vi "MSScript_Act_Execution.vi"(8 "error in (no error)":errorcluster, 11 "MSScript in":refnum<class "MSScript.lvclass">) -> (0 "error out":errorcluster, 3 "MSScript out":refnum<class "MSScript.lvclass">)   [LabVIEW 2018, in "MSScript.lvclass"]
uses:
  MSScript.lvclass
  MSScript.lvclass/MSScript.ctl
  MSScript_Error_(6002)UndefinedSentence.vi
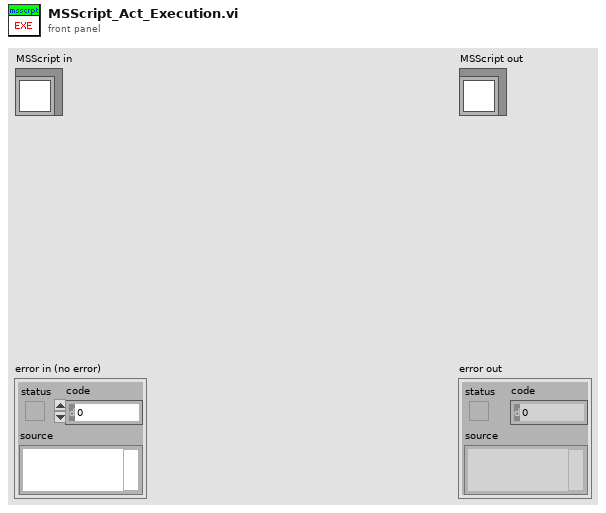
[diagram p1: front panel]
types:
  T1 = cluster{"Type":string, "NAME":cluster{"STR":string, "Start":i32}, "PARAMs":cluster{"STR":string, "Start":i32}[]}[]
  T2 = cluster{"Type":string, "NAME":cluster{"STR":string, "Start":i32}, "PARAMs":cluster{"STR":string, "Start":i32}[]}
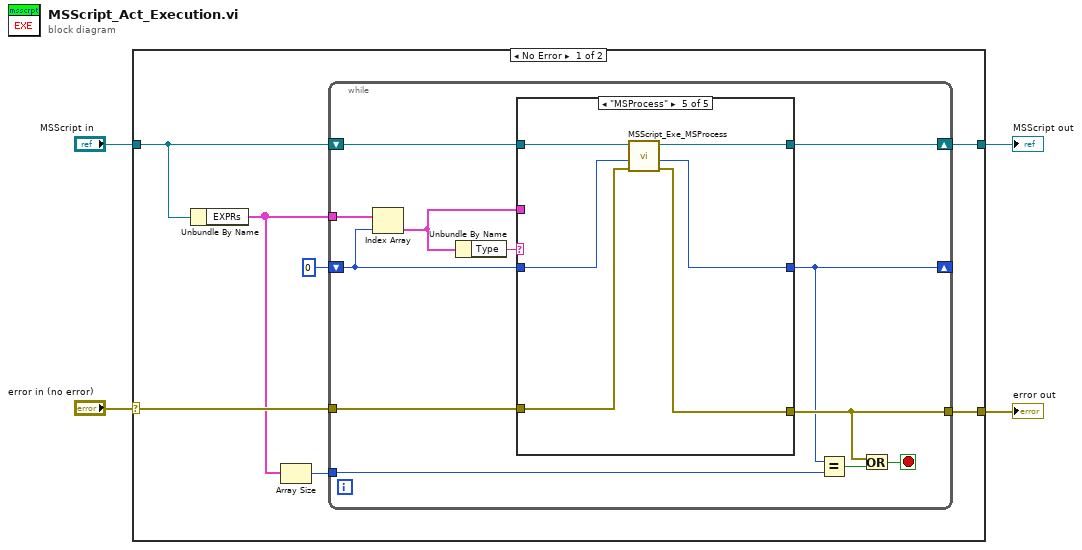
[diagram p0: block diagram]
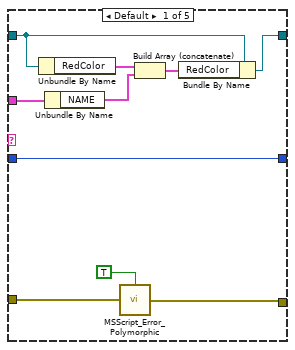
[diagram p2: hidden frame]
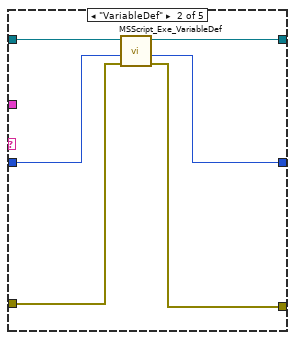
[diagram p3: hidden frame]
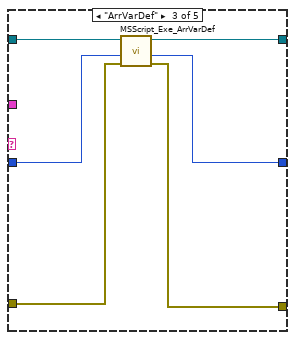
[diagram p4: hidden frame]
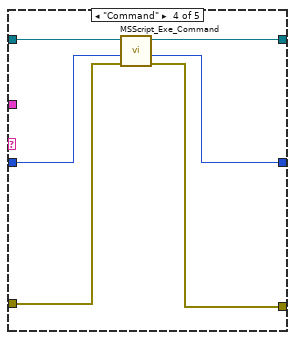
[diagram p5: hidden frame]
diagram:
  n1 = case shown="No Error" "error in (no error)" {
    selector: "error in (no error)" -> [w10 w59]
    tunnel: [w7 w59] -> w3
    tunnel: [w8 w58] -> w1
    tunnel: "MSScript in" -> [w9 w58]
    frame No Error {
      n2 = Unbundle By Name(w9) -> ("EXPRs"=w5:T1)
      n3 = Array Size(array=w5) -> (size(s)=w6:i32)
      n4 = while {
        tunnel: w5 -> [w15]
        shift-right: [w14] -> _
        shift-left: 0 -> [w22]
        tunnel: w10 -> [w21]
        tunnel: [w17] -> w7
        shift-right: [w19] -> w8
        shift-left: w9 -> [w20]
        tunnel: w6 -> [w12]
        stop <- w16 stop-if-true
        n5 = Index Array(array=w15, index=w22) -> (element=w18:T2)
        n6 = Unbundle By Name(w18) -> ("Type"=w23:string)
        n7 = case shown="\"MSProcess\"" w23 {
          tunnel: w22 -> [w32 w37 w43 w47 w56]
          tunnel: w21 -> [w31 w35 w40 w50 w53]
          tunnel: w20 -> [w25 w39 w44 w46 w57]
          tunnel: [w24 w38 w45 w51 w55] -> w19
          tunnel: [w29 w34 w41 w49 w52] -> w17
          tunnel: [w32 w36 w42 w48 w54] -> w14
          tunnel: w18 -> [w33 _ _ _ _]
          frame Default {
            n8 = Unbundle By Name(w25) -> ("RedColor"=w28:cluster{"STR":string, "Start":i32}[])
            n9 = Unbundle By Name(w33) -> ("NAME"=w27:cluster{"STR":string, "Start":i32})
            n10 = call-poly "MSScript_Error_Polymorphic.vi"("error in (no error)"=w31, "ErrBoolean"=TRUE) -> ("error out"=w29:errorcluster)
            n11 = Build Array (concatenate)(w28, w27) -> (w26:cluster{"STR":string, "Start":i32}[])
            n12 = Bundle By Name(cluster=w25, "RedColor"=w26) -> (w24:refnum<class "MSScript.lvclass">)
          }
          frame "VariableDef" {
            n13 = call "MSScript_Exe_VariableDef.vi"("error in (no error)"=w35, "Expression index"=w37, "MSScript in"=w39) -> ("Error out"=w34:errorcluster, "Next expression index"=w36:i32, "MSScript out"=w38:refnum<class "MSScript.lvclass">)  [unwired: 6 in]
          }
          frame "ArrVarDef" {
            n14 = call "MSScript_Exe_ArrVarDef.vi"("error in (no error)"=w40, "Expression index"=w43, "MSScript in"=w44) -> ("Error out"=w41:errorcluster, "Next expression index"=w42:i32, "MSScript out"=w45:refnum<class "MSScript.lvclass">)  [unwired: 6 in]
          }
          frame "Command" {
            n15 = call "MSScript_Exe_Command.vi"("error in (no error)"=w50, "Expression index"=w47, "MSScript in"=w46) -> ("Error out"=w49:errorcluster, "Next expression index"=w48:i32, "MSScript out"=w51:refnum<class "MSScript.lvclass">)  [unwired: 6 in]
          }
          frame "MSProcess" {
            n16 = call "MSScript_Exe_MSProcess.vi"("error in (no error)"=w53, "EXPR Index in"=w56, "MSScript in"=w57) -> ("error out"=w52:errorcluster, "EXPR Index out"=w54:i32, "MSScript out"=w55:refnum<class "MSScript.lvclass">)  [unwired: 6 in]
          }
        }
        n17 = Equal?(x=w14, y=w12) -> (x = y?=w13:bool)
        n18 = Or(x=w17, y=w13) -> (x .or. y?=w16:bool)
      }
    }
    frame Error {
    }
  }
  "error out" <- w3
  "MSScript out" <- w1
